vi "U8翻转(布尔）.vi"(1 "数值":u8) -> (0 "翻转":u8)   [LabVIEW 2012]
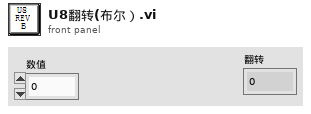
[diagram p1: front panel]
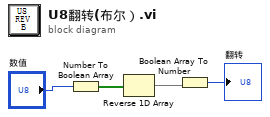
[diagram p0: block diagram]
diagram:
  n1 = Number To Boolean Array(number="数值") -> (Boolean array=w3:bool[])
  n2 = Reverse 1D Array(array=w3) -> (reversed array=w2:bool[])
  n3 = Boolean Array To Number ("布尔数组至数值转换")(Boolean array=w2) -> (number=→"翻转":u8)
